vi "SaveLoadedValues.vi"(0 "Panel Location?":path, 4 "DIMControlSet in":refnum<vi>[](array[refnum])) -> (14 "File Saved?":bool, 17 "File Name":string, 18 "DIMControlSet out":refnum<vi>[](array[refnum]), 19 "Path":path)   [LabVIEW 2014, in "Panels.lvlib"]
uses:
  Panels.lvlib
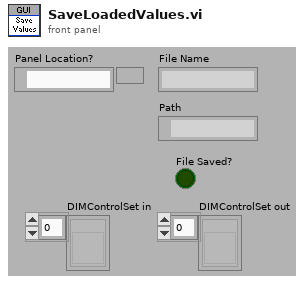
[diagram p1: front panel]
types:
  T1 = cluster{"data":dbl[], "no link":bool, "quality":i32, "timeStamp":dbl}
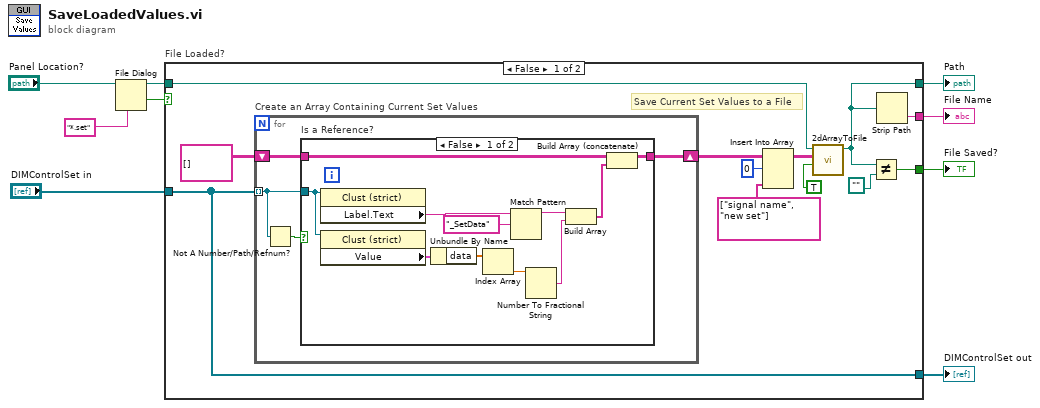
[diagram p0: block diagram]
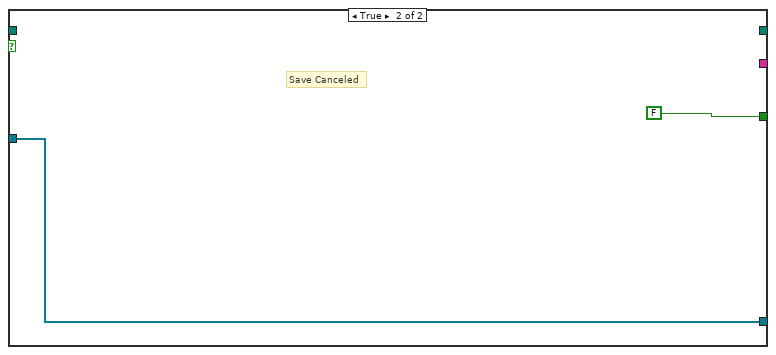
[diagram p3: hidden frame]
diagram:
  n1 = File Dialog(6:"*.set" ("pattern (all files)"), 11:"Panel Location?") -> (1:w8:bool, 3:w9:path)  [unwired: 5 in, 2 out]
  n2 = case "File Loaded?" shown="False" w8 {
    tunnel: w9 -> [w11 _]
    tunnel: "DIMControlSet in" -> [w15 w38]
    tunnel: [w13 FALSE] -> w5
    tunnel: [w16 _] -> w3
    tunnel: [w10 _] -> w2
    tunnel: [w15 w38] -> w1
    frame False {
      # "Save Current Set Values to a File"
      n3 = for "Create an Array Containing Current Set Values" {
        tunnel: w15 -> [w24] mode=indexing
        shift-right: [w23] -> w18
        shift-left: string[][] [] -> [w25]
        n4 = Not A Number/Path/Refnum?(number/path/refnum=w24) -> (NaN/Path/Refnum?=w22:bool)
        n5 = case "Is a Reference?" shown="False" w22 {
          tunnel: w25 -> [w36 w37]
          tunnel: w24 -> [w26 _]
          tunnel: [w35 w37] -> w23
          frame False {
            n6 = property class="Clust (strict)"(reference=w26) -> ("Label.Text"=w31:string)  [unwired: 1 in, 2 out]
            n7 = property class="Clust (strict)"(reference=w26) -> ("Value"=w29:T1)  [unwired: 1 in, 2 out]
            n8 = Unbundle By Name(w29) -> ("data"=w28:dbl[])
            n9 = Index Array(array=w28) -> (element=w27:dbl)  [unwired: 1 in]
            n10 = Match Pattern(string=w31, regular expression="_SetData") -> (before substring=w30:string)  [unwired: 1 in, 3 out]
            n11 = Number To Fractional String(number=w27) -> (F-format string=w33:string)  [unwired: 3 in]
            n12 = Build Array(w30, w33) -> (w34:string[])
            n13 = Build Array (concatenate)(w36, w34) -> (w35:string[][])
          }
          frame True {
          }
        }
      }
      n14 = Insert Into Array(array=w18, index (row)=0, new element=string[] ["signal name", "new set"]) -> (w17:string[][])  [unwired: 1 in]
      n15 = call "2dArrayToFile.vi"("advisory dialog? (display:T)"=TRUE, "Array"=w17, "file path (dialog if empty)"=w11) -> ("new file path (Not A Path if cancelled)"=w10:path)  [unwired: 6 in]
      n16 = Not Equal?(x=w10, y=path "") -> (x != y?=w13:bool)
      n17 = Strip Path(path=w10) -> (name=w16:string)  [unwired: 1 out]
    }
    frame True {
      # "Save Canceled"
    }
  }
  "File Saved?" <- w5
  "File Name" <- w3
  "Path" <- w2
  "DIMControlSet out" <- w1
